vi "TurnOff.vi"(8 "error in (no error)":errorcluster, 11 "PSU_N87 in":refnum<class "PSU_N67.lvclass">) -> (0 "error out":errorcluster, 3 "PSU_N87 out":refnum<class "PSU_N67.lvclass">)   [LabVIEW 2014, in "PSU_N67.lvclass"]
uses:
  PSU_N67.lvclass
  PSU.lvclass/PSU.ctl
  PSU_N67.lvclass/PSU_N67.ctl
  Read Channel.vi
  PSU.lvclass
  data/Agilent N6700 Series.lvlib
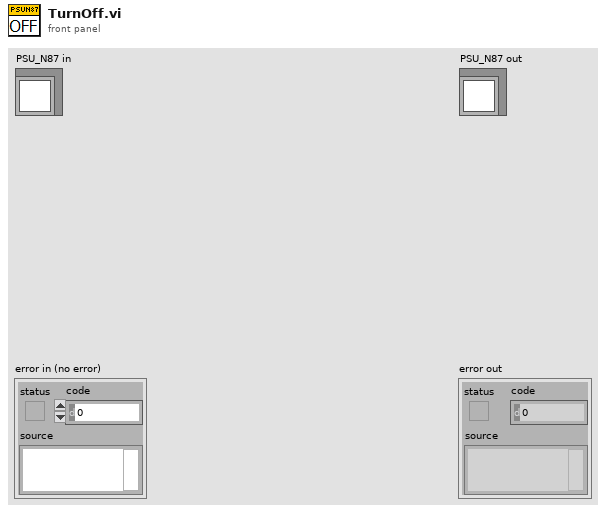
[diagram p1: front panel]
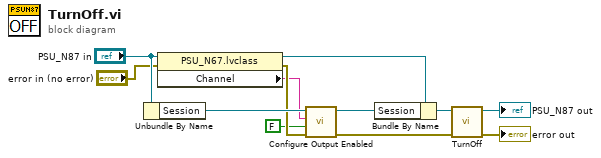
[diagram p0: block diagram]
diagram:
  n1 = Unbundle By Name("PSU_N87 in") -> ("Session"=w11:refnum<visa-resource-name>)
  n2 = property class="PSU_N67.lvclass"(reference="PSU_N87 in", error in="error in (no error)") -> (reference out=w5:refnum<class "PSU_N67.lvclass">, error out=w9:errorcluster, "Channel"=w7:string)
  n3 = call "Configure Output Enabled.vi"("error in (no error)"=w9, "Enable Output (False)"=FALSE, "Channel Name (1)"=w7, "VISA resource name"=w11) -> ("error out"=w2:errorcluster, "VISA resource name out"=w6:refnum<visa-resource-name>)  [unwired: 6 in]
  n4 = Bundle By Name(cluster=w5, "Session"=w6) -> (w4:refnum<class "PSU_N67.lvclass">)
  n5 = call-parent "TurnOff.vi"("error in (no error)"=w2, "PSU in"=w4) -> ("error out"=→"error out":errorcluster, "PSU out"=→"PSU_N87 out":refnum<class "PSU_N67.lvclass">)  [unwired: 8 in]
